vi "FdxCmdTMCreateCvi.vi"(8 "error in":errorcluster, 9 "TMCreateIn":T1, 11 "InstrumentHandle":u32) -> (0 "error out":errorcluster, 2 "TMHandle":u32, 3 "InstrumentHandle Out":u32)   [LabVIEW 2020, in "AIM664LV.lvlib"]
doc: "This function is used to create a Time Manger on a board port. For proper Time\nManager operation, the board must be in redundant mode."
uses:
  AIM664LV.lvlib
  AFDX_LibraryAdmin/FdxGlobalDllPath.vi
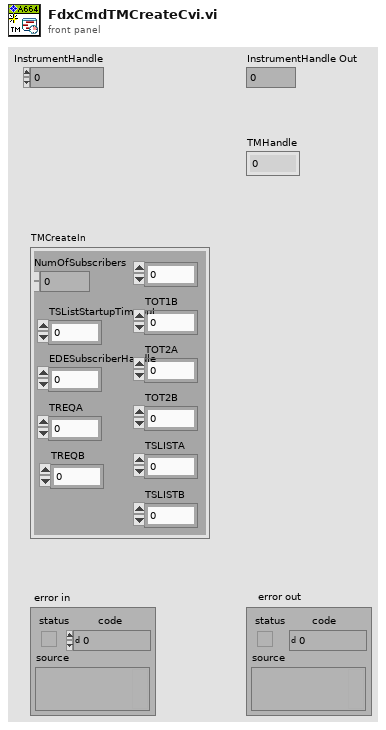
[diagram p1: front panel]
types:
  T1 = cluster{"NumOfSubscribers":u8, "TSListStartupTimeout":u32, "EDESubscriberHandle":u32, "TREQA":u32, "TREQB":u32, "TOT1A":u32, "TOT1B":u32, "TOT2A":u32, "TOT2B":u32, "TSLISTA":u32, "TSLISTB":u32}
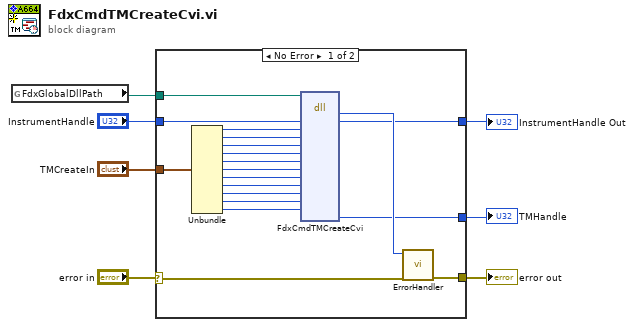
[diagram p0: block diagram]
diagram:
  n1 = global read "FdxGlobalDllPath.vi" "FdxGlobalDllPath"() -> (w5:path)
  n2 = case shown="No Error" "error in" {
    selector: "error in" -> [w25 w28]
    tunnel: [w26 w28] -> w7
    tunnel: w5 -> [w12 _]
    tunnel: "InstrumentHandle" -> [w11 w27]
    tunnel: [w10 w27] -> w3
    tunnel: "TMCreateIn" -> [w9 _]
    tunnel: [w8 _] -> w1
    frame No Error {
      n3 = Unbundle(w9) -> ("NumOfSubscribers"=w23:u8, "TSListStartupTimeout"=w22:u32, "EDESubscriberHandle"=w21:u32, "TREQA"=w20:u32, "TREQB"=w19:u32, "TOT1A"=w18:u32, "TOT1B"=w17:u32, "TOT2A"=w16:u32, "TOT2B"=w15:u32, "TSLISTA"=w14:u32, "TSLISTB"=w13:u32)
      n4 = dll-call lib="aim_fdx.19.dll" fn="FdxCmdTMCreateCvi"(path in=w12, "InstrumentHandle"=w11, "NumberofSubscribers"=w23, "TSListStartupTimeout"=w22, "EDESubscribersHandle"=w21, "TREQA"=w20, "TREQB"=w19, "TOT1A"=w18, "TOT1B"=w17, "TOT2A"=w16, "TOT2B"=w15, "TSLISTA"=w14, "TSLISTB"=w13) -> ("status"=w24:i32, "InstrumentHandle"=w10:u32, "TMHandle"=w8:u32)  [unwired: 13 in, 3 out]
      n5 = call "ErrorHandler.vi"("error in"=w25, "AIM Error"=w24) -> ("error out"=w26:errorcluster)  [unwired: 9 in]
    }
    frame Error {
    }
  }
  "error out" <- w7
  "InstrumentHandle Out" <- w3
  "TMHandle" <- w1
